vi "Status.vi"(7 "Mode":T1=enum."Testing", 8 "error in (no error)":errorcluster, 11 "Data":bool) -> (0 "error out":errorcluster, 2 "Testing":bool, 3 "Connections":cluster{"Data":bool, "Data":bool, "Data":bool})   [LabVIEW 2016]
uses:
  Controls/staus modes.ctl
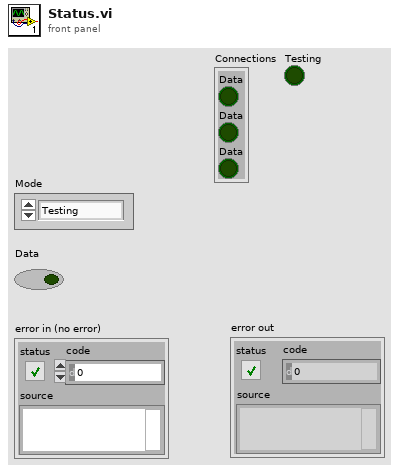
[diagram p1: front panel]
types:
  T1 = typedef "staus modes.ctl" = enum16{"Status", "Testing", "Webcam", "DAQ", "Actuator", "Initialise"}
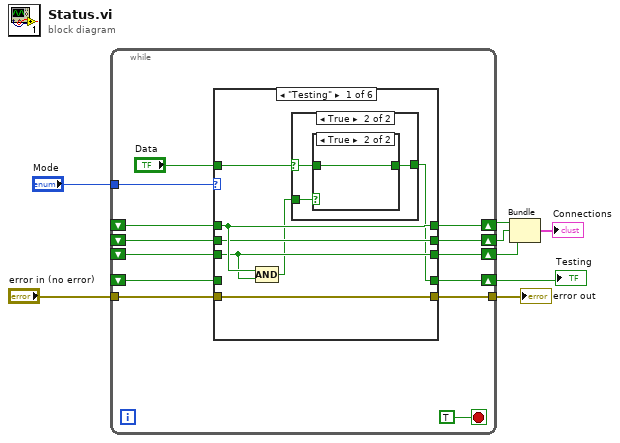
[diagram p0: block diagram]
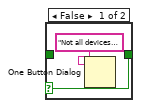
[diagram p3: hidden frame]
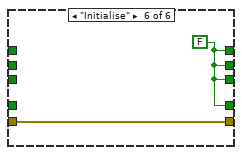
[diagram p8: hidden frame]
diagram:
  n1 = while {
    tunnel: "Mode" -> [w20]
    tunnel: "error in (no error)" -> [w19]
    tunnel: [w18] -> w6
    shift-right: [w14] -> w5
    shift-left: _ -> [w15]
    shift-right: [w13] -> w4
    shift-left: _ -> [w10]
    shift-right: [w12] -> w3
    shift-left: _ -> [w9]
    shift-right: [w11] -> w1
    shift-left: _ -> [w16]
    stop <- TRUE stop-if-true
    n2 = case shown="\"Testing\"" w20 {
      tunnel: w19 -> [w28 w36 w45 w46 w51 w56]
      tunnel: [w28 w36 w45 w46 w51 w56] -> w18
      tunnel: "Data" -> [w24 _ w44 w48 w55 _]
      tunnel: w16 -> [_ w37 w41 w47 w52 _]
      tunnel: w15 -> [w27 w40 w43 w50 _ _]
      tunnel: [w27 w40 w43 w50 w55 w57] -> w14
      tunnel: [w26 w39 w44 w49 w54 w57] -> w13
      tunnel: [w25 w38 w42 w48 w53 w57] -> w12
      tunnel: [w22 w37 w41 w47 w52 w57] -> w11
      tunnel: w10 -> [w26 w39 _ w49 w54 _]
      tunnel: w9 -> [w25 w38 w42 _ w53 _]
      frame "Testing" {
        n3 = Compound Arithmetic op=AND(w27, w25) -> (w23:bool)
        n4 = case shown="True" w24 {
          selector: w24 -> [w29 w31]
          tunnel: w23 -> [_ w32]
          tunnel: [w29 w30] -> w22
          frame False {
          }
          frame True {
            n5 = case shown="True" w32 {
              selector: w32 -> [w33 _]
              tunnel: w31 -> [_ w35]
              tunnel: [w33 w35] -> w30
              frame False {
                n6 = One Button Dialog(message="Not all devices connected") -> ()  [unwired: 1 in, 1 out]
              }
              frame True {
              }
            }
          }
        }
      }
      frame "Status", Default {
      }
      frame "Webcam" {
      }
      frame "DAQ" {
      }
      frame "Actuator" {
      }
      frame "Initialise" {
        w57 = FALSE
      }
    }
  }
  "error out" <- w6
  "Testing" <- w1
  n7 = Bundle("Data"=w5, "Data"=w4, "Data"=w3) -> (→"Connections":cluster{"Data":bool, "Data":bool, "Data":bool})  [unwired: 1 in]
